vi "exercise1_firstvi.vi"(11 "angulo grados":dbl) -> ()   [LabVIEW 2018]
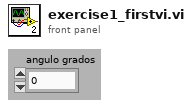
[diagram p1: front panel]
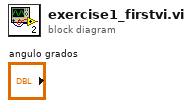
[diagram p0: block diagram]
diagram:
